vi "基础11.vi"() -> ()   [LabVIEW 2014]
panel:
  out "字符串":string
  in  "数值":dbl
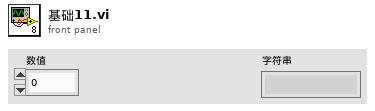
[diagram p1: front panel]
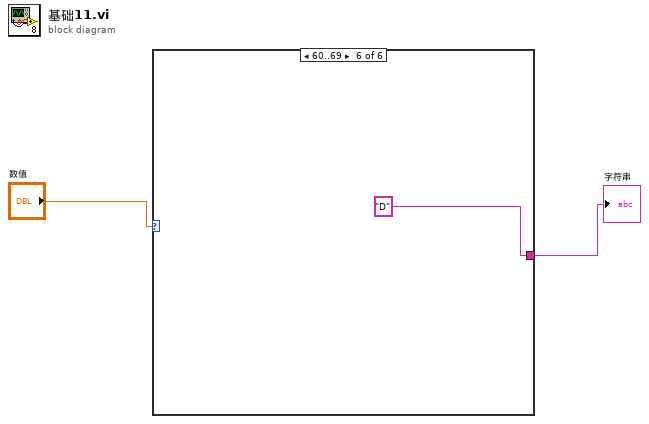
[diagram p0: block diagram]
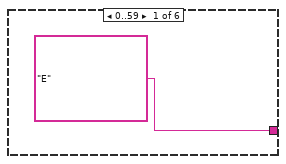
[diagram p2: hidden frame]
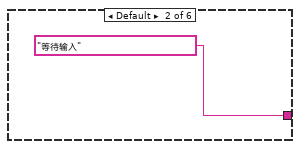
[diagram p3: hidden frame]
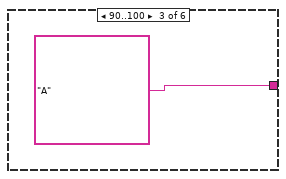
[diagram p4: hidden frame]
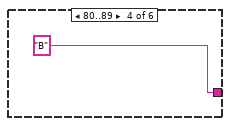
[diagram p5: hidden frame]
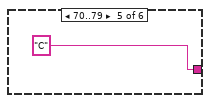
[diagram p6: hidden frame]
diagram:
  n1 = case shown="60..69" "数值" {
    tunnel: ["E" "等待输入" "A" "B" "C" "D"] -> w1
    frame 0..59 {
    }
    frame Default {
    }
    frame 90..100 {
    }
    frame 80..89 {
    }
    frame 70..79 {
    }
    frame 60..69 {
    }
  }
  "字符串" <- w1
